vi "AddTiffPage_U16_text.vi"(0 "TIFF file":T1 {"BigTiff,Endian" items=["Big-Endian"=0, "Native"=1, "Little-Endian"=2, "BigTiff-Big-Endian"=256, "Bigtiff,Native"=257, "Biftiff,Littleendian"=258]}, 1 "After last DIROffset":u64=8, 2 "Text":string="test", 3 "16-bit pixmap x, y":u16[][](array[numeric])) -> (5 "TIFF file":T1 {"BigTiff,Endian" items=["Big-Endian"=0, "Native"=1, "Little-Endian"=2, "BigTiff-Big-Endian"=256, "Bigtiff,Native"=257, "Biftiff,Littleendian"=258]}, 6 "AfterDIRoffset":u64 format="%.0x", 7 "error out":errorcluster)   [LabVIEW 2011]
panel:
  out "IFD-Offste written":i64 format="%.0x"
  in  "error in":errorcluster
  out "eof\nstart here":i64
  out "size(s)":i32[](array[numeric])
  out "Directory Entries":T2(array[cluster])
  # "the 4/8 bytes before will be changed"
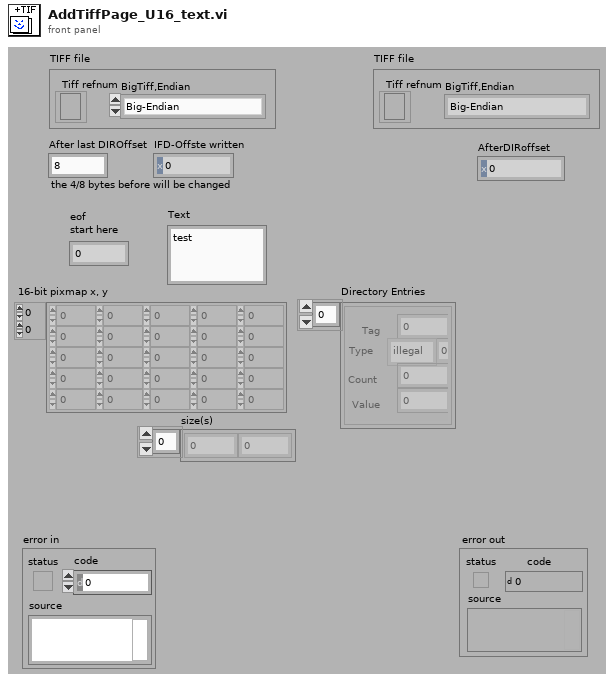
[diagram p1: front panel]
types:
  T1 = cluster{"Tiff refnum":refnum<file>, "BigTiff,Endian":u16}
  T2 = cluster{"Tag":u16, "Type":enum16{"illegal", "Byte", "Ascii", "Short", "Long"}, "Count":u32, "Value":u32}[]
  T3 = typedef "IFD.ctl" = cluster{"Tag":u16, "Type":enum16{"illegal", "Byte", "Ascii", "Short", "Long", "Rational", "SByte", "Undefined", "SShort", "SLong", "SRational 2xSLong", "Float 4byte", "Double 8Byte", "No13", "No14", "No15", "U64", "I64", "U64-IFD8"}, "Count":u64, "Value":u64}
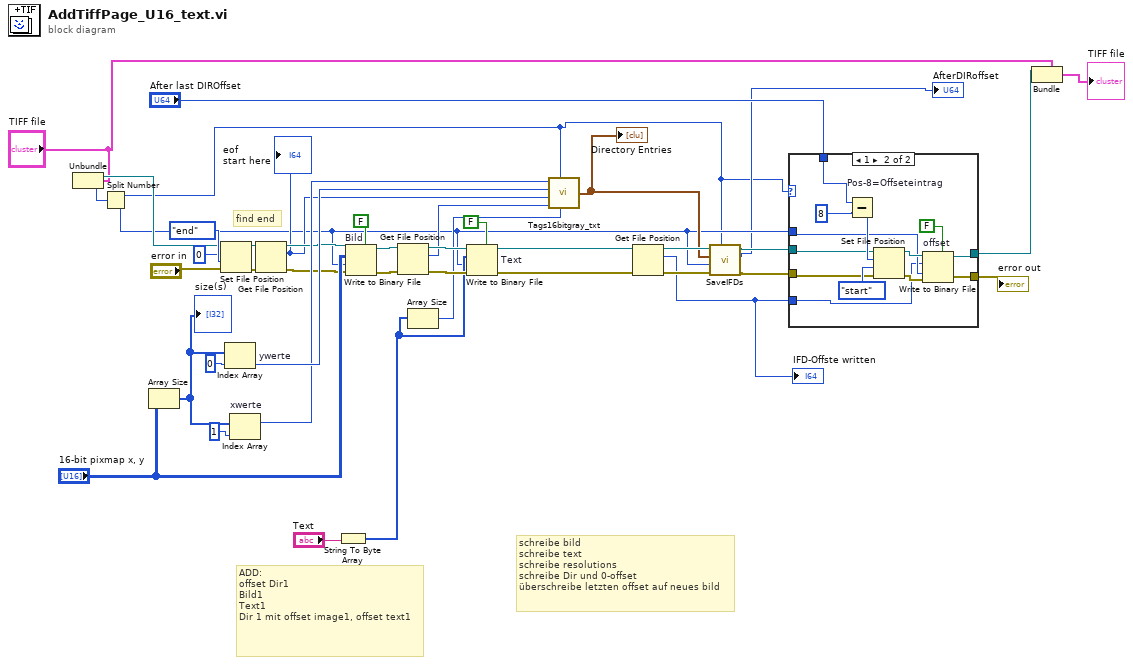
[diagram p0: block diagram]
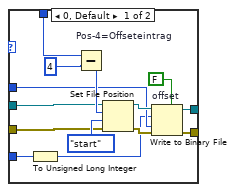
[diagram p2: hidden frame]
diagram:
  # "find end"
  # "schreibe bild\nschreibe text\nschreibe resolutions\nschreibe Dir und 0-offset\nüberschreibe letzten offset auf neues bild"
  # "ADD:\noffset Dir1\nBild1\nText1\nDir 1 mit offset image1, offset text1"
  n1 = Unbundle("TIFF file") -> ("Tiff refnum"=w23:refnum<file>, "BigTiff,Endian"=w10:u16)
  n2 = Split Number(x=w10) -> (hi(x)=w1:u8, lo(x)=w6:u8)
  n3 = Array Size(array="16-bit pixmap x, y") -> (size(s)=w40:i32[])
  "size(s)" <- w40
  n4 = Set File Position(offset (in bytes) (0)=0 ("pos offset (0)"), refnum=w23, from (0:start)=enum16{"start", "end", "current"}."end" ("pos mode (0:2)"), error in="error in") -> (refnum out=w31:refnum<file>, error out=w30:errorcluster)
  n5 = Index Array "ywerte"(array=w40, index=0 ("Index")) -> (element=w39:i32)
  n6 = Index Array "xwerte"(array=w40, index=1 ("Index")) -> (element=w38:i32)
  n7 = Get File Position(4:w30, 7:w31) -> (0:w21:errorcluster, 2:w17:i64, 3:w22:refnum<file>)
  "eof\nstart here" <- w17
  n8 = String To Byte Array(string="Text") -> (unsigned byte array=w12:u8[])
  n9 = Write to Binary File "Bild"(file (use dialog)=w22, data="16-bit pixmap x, y", error in=w21, 5:FALSE ("Array- oder Stringgröße voranstellen? (T)"), 9:w6) -> (refnum out=w26:refnum<file>, error out=w25:errorcluster)  [unwired: 2 out]
  n10 = Get File Position(4:w25, 7:w26) -> (0:w20:errorcluster, 2:w18:i64, 3:w19:refnum<file>)
  n11 = Array Size(array=w12) -> (size(s)=w11:i32)
  n12 = Write to Binary File "Text"(file (use dialog)=w19, data=w12, error in=w20, 5:FALSE ("Array- oder Stringgröße voranstellen? (T)"), 9:w6) -> (refnum out=w29:refnum<file>, error out=w28:errorcluster)  [unwired: 2 out]
  n13 = call "Tags16bitgray_txt.vi"("xbreite"=w38, "BigTiff"=w1, "yhöhe"=w39, "BildOffset Bytes"=w17, "Text length"=w11, "Text Offset Bytes"=w18) -> ("Directory Entrys"=w7:T3[])  [unwired: 2 out]
  "Directory Entries" <- w7
  n14 = Get File Position(4:w28, 7:w29) -> (0:w9:errorcluster, 2:w2:i64, 3:w8:refnum<file>)
  "IFD-Offste written" <- w2
  n15 = call "SaveIFDs.vi"("BigTiff"=w1, "Fehler (Eingang)"=w9, "Byte-Reihenfolge (0:Big-Endian, Netzwerkreihenfolge)"=w6, "IFDs"=w7, "Refnum"=w8) -> ("Fehler (Ausgang)"=w4:errorcluster, "after next offset (zero)"=→"AfterDIRoffset":i64, "Refnum (Ausgang)"=w5:refnum<file>)  [unwired: 4 out]
  n16 = case shown="1" w1 {
    tunnel: "After last DIROffset" -> [w53 w57]
    tunnel: [w52 w58] -> w32
    tunnel: [w48 w59] -> w16
    tunnel: w6 -> [w47 w63]
    tunnel: w5 -> [w46 w62]
    tunnel: w4 -> [w45 w61]
    tunnel: w2 -> [w44 w60]
    frame 0, Default {
      n17 = To Unsigned Long Integer(number=w44) -> (unsigned 32bit integer=w43:u32)
      n18 = Subtract "Pos-4=Offseteintrag"(x=w53, y=u32 4) -> (x-y=w54:u64)
      n19 = Set File Position(offset (in bytes) (0)=w54, refnum=w46, from (0:start)=enum16{"start", "end", "current"}."start" ("pos mode (0:2)"), error in=w45) -> (refnum out=w51:refnum<file>, error out=w50:errorcluster)
      n20 = Write to Binary File "offset"(file (use dialog)=w51, data=w43, error in=w50, 5:FALSE ("Array- oder Stringgröße voranstellen? (T)"), 9:w47) -> (refnum out=w48:refnum<file>, error out=w52:errorcluster)  [unwired: 2 out]
    }
    frame 1 {
      n21 = Subtract "Pos-8=Offseteintrag"(x=w57, y=u32 8) -> (x-y=w67:u64)
      n22 = Set File Position(offset (in bytes) (0)=w67, refnum=w62, from (0:start)=enum16{"start", "end", "current"}."start" ("pos mode (0:2)"), error in=w61) -> (refnum out=w66:refnum<file>, error out=w65:errorcluster)
      n23 = Write to Binary File "offset"(file (use dialog)=w66, data=w60, error in=w65, 5:FALSE ("Array- oder Stringgröße voranstellen? (T)"), 9:w63) -> (refnum out=w59:refnum<file>, error out=w58:errorcluster)  [unwired: 2 out]
    }
  }
  "error out" <- w32
  n24 = Bundle(cluster="TIFF file", "Tiff refnum"=w16) -> (→"TIFF file":T1)  [unwired: 1 out]
